vi "Get Orientation.vi"(1 "Component.lvclass":refnum<class "Component.lvclass">) -> (0 "landscape?":bool)   [LabVIEW 2023, in "Component.lvclass"]
doc: "Get this component's rotational orientation."
uses:
  Component.lvclass
  Component.lvclass/Component.ctl
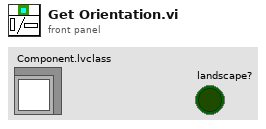
[diagram p1: front panel]
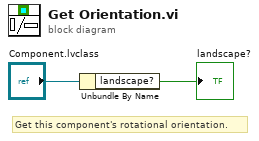
[diagram p0: block diagram]
diagram:
  # "Get this component's rotational orientation."
  n1 = Unbundle By Name("Component.lvclass") -> ("landscape?"=→"landscape?":bool)
